vi "contolador de variables.vi"(8 "CONTROL DE LLENADO":cluster{"SET POINT":dbl, "INC  L":dbl}, 9 "CONTROL DE HUMEDAD":cluster{"SET POINT":dbl, "INC %":dbl}, 10 "CONTROL DE PRESIÓN":cluster{"SET POINT":dbl, "INC P":dbl}, 11 "CONTROL TEMPERATURA":cluster{"SET POINT":dbl, "INC T":dbl}) -> (0 "VOLUMEN ACTUAL":dbl, 1 "HUMEDAD ACTUAL":dbl, 2 "PRESIÓN ACTUAL":dbl, 3 "TEMPERATURA ACTUAL":dbl)   [LabVIEW 2017]
doc: "Simula un sistema de control para cuatro variables (Temperatura, Presión, Humedad y Volumen). Para efectuar el control de una variable hay que especificar el valor objetivo (set point) y el incremento de valor por cada ejecución."
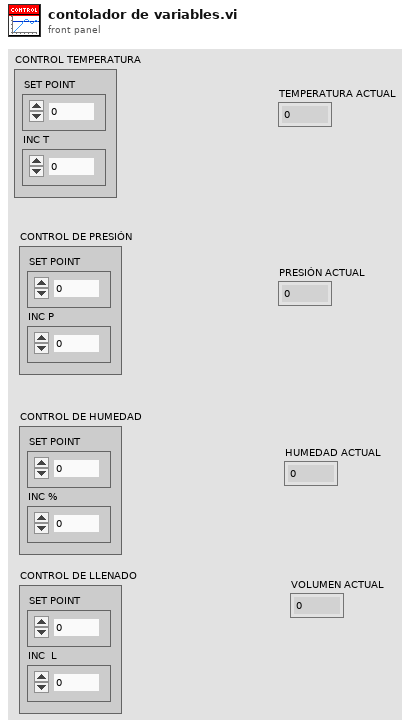
[diagram p1: front panel]
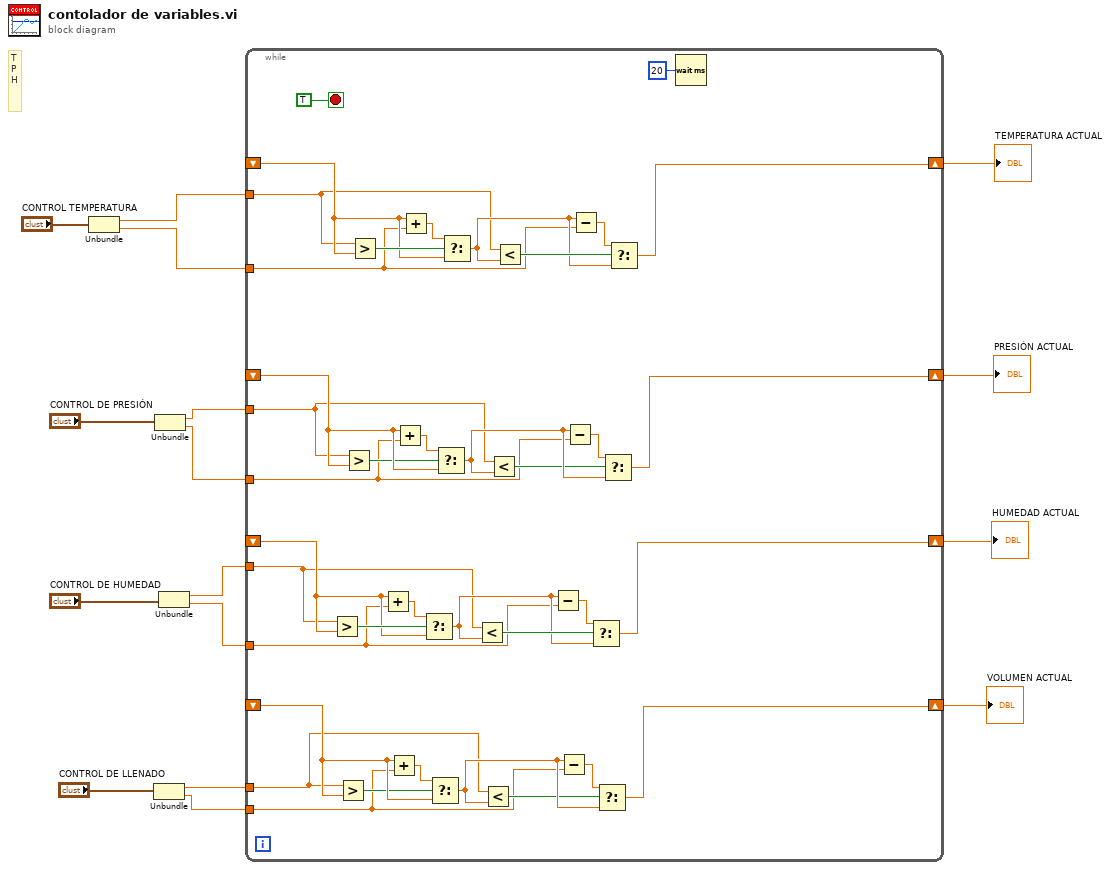
[diagram p0: block diagram]
diagram:
  # "T\nP\nH"
  n1 = Unbundle("CONTROL TEMPERATURA") -> ("SET POINT"=w11:dbl, "INC T"=w10:dbl)
  n2 = Unbundle("CONTROL DE LLENADO") -> ("SET POINT"=w2:dbl, "INC  L"=w1:dbl)
  n3 = Unbundle("CONTROL DE PRESIÓN") -> ("SET POINT"=w8:dbl, "INC P"=w7:dbl)
  n4 = Unbundle("CONTROL DE HUMEDAD") -> ("SET POINT"=w5:dbl, "INC %"=w4:dbl)
  n5 = while {
    shift-right: [w49] -> w16
    shift-left: _ -> [w50]
    shift-right: [w45] -> w13
    shift-left: _ -> [w44]
    shift-right: [w34] -> w14
    shift-left: _ -> [w35]
    shift-right: [w31] -> w15
    shift-left: _ -> [w30]
    tunnel: w11 -> [w24]
    tunnel: w10 -> [w23]
    tunnel: w8 -> [w22]
    tunnel: w7 -> [w21]
    tunnel: w5 -> [w20]
    tunnel: w4 -> [w19]
    tunnel: w2 -> [w18]
    tunnel: w1 -> [w17]
    stop <- TRUE stop-if-true
    n6 = Greater?(x=w20, y=w35) -> (0:w39:bool)
    n7 = Greater?(x=w18, y=w30) -> (0:w26:bool)
    n8 = Greater?(x=w22, y=w44) -> (0:w40:bool)
    n9 = Greater?(x=w24, y=w50) -> (0:w54:bool)
    n10 = Add(x=w35, y=w19) -> (x+y=w38:dbl)
    n11 = Add(x=w30, y=w17) -> (x+y=w27:dbl)
    n12 = Add(x=w44, y=w21) -> (x+y=w41:dbl)
    n13 = Add(x=w50, y=w23) -> (x+y=w53:dbl)
    n14 = Select(t=w38, s=w39, f=w35) -> (s? t:f=w33:dbl)
    n15 = Select(t=w27, s=w26, f=w30) -> (s? t:f=w32:dbl)
    n16 = Select(t=w41, s=w40, f=w44) -> (s? t:f=w46:dbl)
    n17 = Select(t=w53, s=w54, f=w50) -> (s? t:f=w47:dbl)
    n18 = Less?(x=w20, y=w33) -> (x < y?=w37:bool)
    n19 = Less?(x=w18, y=w32) -> (x < y?=w28:bool)
    n20 = Less?(x=w22, y=w46) -> (x < y?=w42:bool)
    n21 = Less?(x=w24, y=w47) -> (x < y?=w52:bool)
    n22 = Subtract(x=w33, y=w19) -> (x-y=w36:dbl)
    n23 = Subtract(x=w32, y=w17) -> (x-y=w29:dbl)
    n24 = Subtract(x=w46, y=w21) -> (x-y=w43:dbl)
    n25 = Subtract(x=w47, y=w23) -> (x-y=w51:dbl)
    n26 = Select(t=w36, s=w37, f=w33) -> (s? t:f=w34:dbl)
    n27 = Select(t=w29, s=w28, f=w32) -> (s? t:f=w31:dbl)
    n28 = Select(t=w43, s=w42, f=w46) -> (s? t:f=w45:dbl)
    n29 = Select(t=w51, s=w52, f=w47) -> (s? t:f=w49:dbl)
    n30 = Wait (ms)(milliseconds to wait=u32 20) -> ()  [unwired: 1 out]
  }
  "TEMPERATURA ACTUAL" <- w16
  "PRESIÓN ACTUAL" <- w13
  "HUMEDAD ACTUAL" <- w14
  "VOLUMEN ACTUAL" <- w15
